vi "CorrectALLTDMS_HBM_Files.vi"() -> ()   [LabVIEW 2017]
panel:
  out "Numérique":i32
  out "sortie d'erreur":errorcluster
  out "error out":errorcluster
  out "chemin complet":path
  in  "entrée d'erreur":errorcluster
  in  "chemin":path
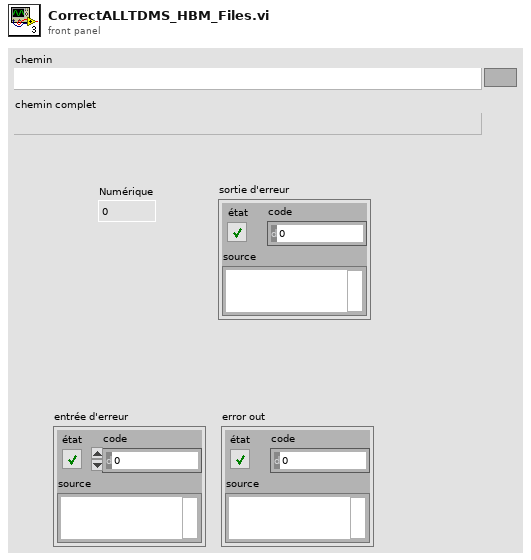
[diagram p1: front panel]
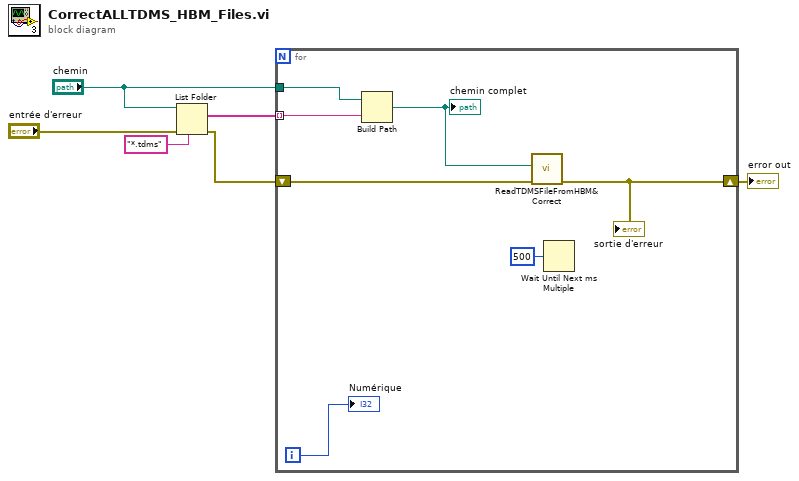
[diagram p0: block diagram]
diagram:
  n1 = List Folder(path="chemin", pattern="*.tdms" ("filtre"), error in="entrée d'erreur") -> (filenames=w5:string[], error out=w3:errorcluster)  [unwired: 1 in, 2 out]
  n2 = for {
    tunnel: w5 -> [w12] mode=indexing
    tunnel: "chemin" -> [w13]
    shift-right: [w9] -> w1
    shift-left: w3 -> [w10]
    i -> [w7]
    n3 = Build Path(base path=w13, name or relative path=w12) -> (appended path=w8:path)
    "chemin complet" <- w8
    n4 = call "ReadTDMSFileFromHBM&Correct.vi"("error in (no error)"=w10, "file path"=w8) -> ("sortie d'erreur"=w9:errorcluster)  [unwired: 4 in, 1 out]
    "sortie d'erreur" <- w9
    n5 = Wait Until Next ms Multiple(millisecond multiple=u32 500 ("n millisecondes")) -> ()  [unwired: 1 out]
    "Numérique" <- w7
  }
  "error out" <- w1
